vi "ElapsedTime2.vi"(8 "error in (no error)":errorcluster, 10 "Mode (Update)":enum16{"Update", "Init"}(ring)) -> (0 "error out":errorcluster, 2 "Elapsed Time":u32)   [LabVIEW 2013]
doc: "Use this template to build a VI to use as a subVI."
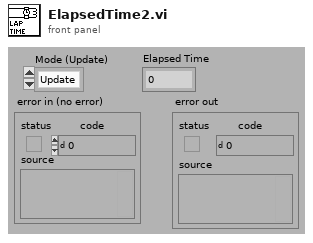
[diagram p1: front panel]
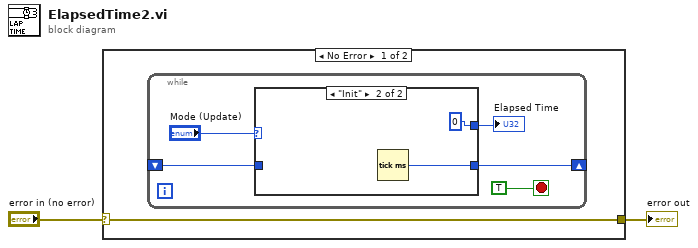
[diagram p0: block diagram]
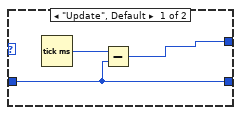
[diagram p2: hidden frame]
diagram:
  n1 = case shown="No Error" "error in (no error)" {
    selector: "error in (no error)" -> [w3 w14]
    tunnel: [w3 w14] -> w1
    frame No Error {
      n2 = while {
        shift-right: [w7] -> _
        shift-left: _ -> [w6]
        stop <- TRUE stop-if-true
        n3 = case shown="\"Init\"" "Mode (Update)" {
          tunnel: w6 -> [w10 _]
          tunnel: [w10 w13] -> w7
          tunnel: [w9 u32 0] -> w5
          frame "Update", Default {
            n4 = Tick Count (ms)() -> (millisecond timer value=w11:u32)
            n5 = Subtract(x=w11, y=w10) -> (x-y=w9:u32)
          }
          frame "Init" {
            n6 = Tick Count (ms)() -> (millisecond timer value=w13:u32)
          }
        }
        "Elapsed Time" <- w5
      }
    }
    frame Error {
    }
  }
  "error out" <- w1
